vi "generate Ic distribution.vi"(5 "gmode":enum16{"TA", "MQT", "TA+MQT"}(ring), 7 "progress indicator":refnum<vi>, 8 "error in (no error)":errorcluster, 10 "Parameters":T1={"temperature K"=0.01, "C0 capacitance F"=0.0, "Ic A"=0.0, "R Ohm"=0.0, "Parity Mode"=enum."No parity", "Parity switch fre"=0.0, "Parity ratio"=0.0, "Imax A"=0.0, "Tsw s"=0.0, "N_steps"=0, "Ic_d"=0.0, "N_sweeps"=0, "Ic_cut"=0.0} {"temperature K" step=0.01}, 11 "path in":path) -> (0 "error out":errorcluster, 2 "return type":dbl[](array[numeric]), 3 "path out":path)   [LabVIEW 2023]
uses:
  paramaters2.ctl
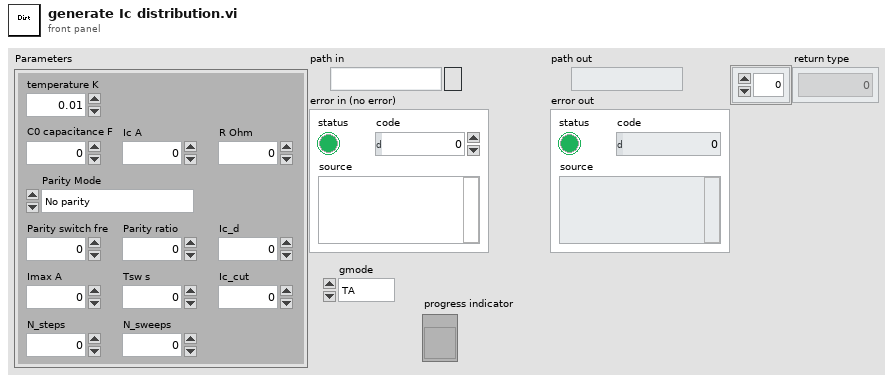
[diagram p1: front panel]
types:
  T1 = typedef "paramaters2.ctl" = cluster{"temperature K":dbl, "C0 capacitance F":dbl, "Ic A":dbl, "R Ohm":dbl, "Parity Mode":enum16{"No parity", "Parity with random lifetime", "For Ic-Ic_d/2", "For Ic+Ic_d/2", "Parity with constant lifetime"}, "Parity switch fre":dbl, "Parity ratio":dbl, "Imax A":dbl, "Tsw s":dbl, "N_steps":i32, "Ic_d":dbl, "N_sweeps":i32, "Ic_cut":dbl}
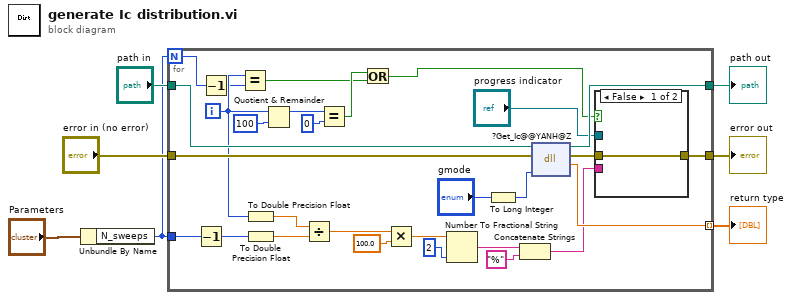
[diagram p0: block diagram]
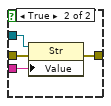
[diagram p2: hidden frame]
diagram:
  n1 = Unbundle By Name("Parameters") -> ("N_sweeps"=w1:i32)
  n2 = for {
    N: w1 -> [w10]
    tunnel: "path in" -> [w36]
    tunnel: [w35] -> w6
    tunnel: "error in (no error)" -> [w34]
    tunnel: [w30] -> w4
    tunnel: [w33] -> w3 mode=indexing
    tunnel: w1 -> [w29]
    i -> [w11]
    n3 = Decrement(x=w29) -> (x-1=w28:i32)
    n4 = Decrement(x=w10) -> (x-1=w8:i32)
    n5 = Equal?(x=w11, y=w8) -> (x = y?=w9:bool)
    n6 = To Double Precision Float(number=w11) -> (double precision float=w27:dbl)
    n7 = To Double Precision Float(number=w28) -> (double precision float=w26:dbl)
    n8 = Quotient & Remainder(x=w11, y=100) -> (x-y*floor(x/y)=w15:i32)  [unwired: 1 out]
    n9 = Divide(x=w27, y=w26) -> (x/y=w25:dbl)
    n10 = Equal?(x=w15, y=0) -> (x = y?=w13:bool)
    n11 = Or(x=w13, y=w9) -> (x .or. y?=w12:bool)
    n12 = Multiply(x=w25, y=100.0) -> (x*y=w22:dbl)
    n13 = Number To Fractional String(number=w22, precision (6)=i16 2) -> (F-format string=w21:string)  [unwired: 2 in]
    n14 = To Long Integer(number="gmode") -> (32bit integer=w17:i32)
    n15 = Concatenate Strings(w21, "%" ("string")) -> (w19:string)
    n16 = dll-call lib="C:/Users/Guang Yue/Desktop/JJ-diffraction-simulation-GUI/ygDLL.dll" fn="?Get_Ic@@YANH@Z"(path in=w36, error in=w34, "gmode"=w17) -> (path out=w35:path, error out=w31:errorcluster, "return type"=w33:dbl)  [unwired: 2 in]
    n17 = case shown="False" w12 {
      tunnel: "progress indicator" -> [_ w41]
      tunnel: w31 -> [w37 w40]
      tunnel: [w37 w39] -> w30
      tunnel: w19 -> [_ w38]
      frame False {
      }
      frame True {
        n18 = property class="Str"(reference=w41, error in=w40, "Value"=w38) -> (error out=w39:errorcluster)  [unwired: 1 out]
      }
    }
  }
  "path out" <- w6
  "error out" <- w4
  "return type" <- w3
